vi "Extreme Value Moments.vi"(9 "b":dbl=1.0, 10 "a":dbl) -> (0 "error":i32, 2 "variance":dbl=1.6449340668482264, 3 "mean":dbl=0.57722)   [LabVIEW 2020, in "NI_Gmath.lvlib"]
doc: "Returns the expected mean and variance of the random variate X, where X describes the selected distribution type. You must manually select the polymorphic instance to use."
uses:
  <vilib>/gmath/NI_Gmath.lvlib
  <vilib>/gmath/statdist.llb/st_error_code.ctl
panel:
  # "Extreme Value Moments"
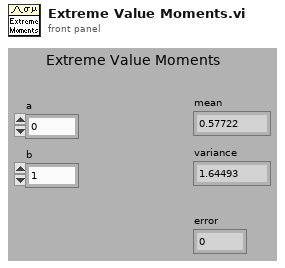
[diagram p1: front panel]
types:
  T1 = typedef "NI_Gmath.lvlib/st_error_code.ctl" = i32
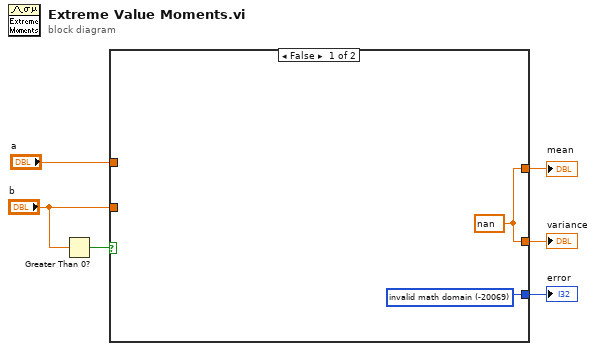
[diagram p0: block diagram]
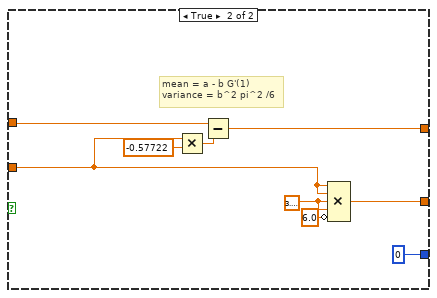
[diagram p2: hidden frame]
diagram:
  n1 = Greater Than 0?(x="b") -> (x > 0?=w6:bool)
  n2 = case shown="False" w6 {
    tunnel: [w7 0 ("invalid math domain")] -> w3
    tunnel: [w8 w9] -> w5
    tunnel: [w8 w13] -> w4
    tunnel: "a" -> [_ w16]
    tunnel: "b" -> [_ w12]
    frame False {
      w7 = T1 -20069 items=["invalid math domain"=-20069, "Fourier interpolation size m >= n"=-20070, "empty array"=-20003] ("stat interp error code")
      w8 = nan
    }
    frame True {
      w11 = 3.141592653589793
      # "mean = a - b G'(1)\nvariance = b^2 pi^2 /6"
      n3 = Multiply(x=w12, y=-0.57722) -> (x*y=w14:dbl)
      n4 = Subtract(x=w16, y=w14) -> (x-y=w13:dbl)
      n5 = Compound Arithmetic op=MULTIPLY(w12, w12, w11, w11, invert 6.0 ("value")) -> (w9:dbl)
    }
  }
  "mean" <- w4
  "error" <- w3
  "variance" <- w5
